vi "获取一个图像区域每一列亮度平均值.vi"(10 "矩形框":dbl[](array[numeric]), 11 "引用句柄输入":T1) -> (3 "数组":dbl[](array[numeric]))   [LabVIEW 2014]
uses:
  <vilib>/vision/Image Controls.llb/IMAQ Image.ctl
  <vilib>/Analysis/baseanly.llb/Mean (DBL).vi
  <vilib>/Analysis/NI_AALBase.lvlib
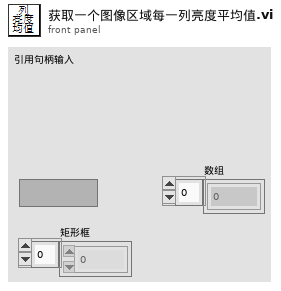
[diagram p1: front panel]
types:
  T1 = typedef "IMAQ Image.ctl" = refnum<image>
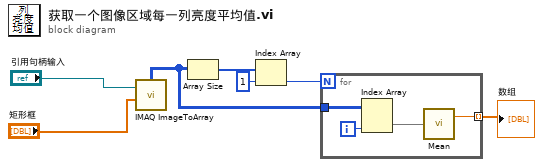
[diagram p0: block diagram]
diagram:
  n1 = call "IMAQ ImageToArray"("Optional Rectangle"="矩形框", "Image"="引用句柄输入") -> ("Image Pixels (U8)"=w1:u8[][])  [unwired: 2 in, 4 out]
  n2 = Array Size(array=w1) -> (size(s)=w2:i32[])
  n3 = Index Array(array=w2, index=1 ("索引")) -> (element=w3:i32)
  n4 = for {
    N: w3 -> [_]
    tunnel: w1 -> [w11]
    tunnel: [w8] -> w5 mode=indexing
    i -> [w10]
    n5 = Index Array(array=w11, index (col)=w10) -> (element=w9:u8[])  [unwired: 1 in]
    n6 = call-poly <vilib>:"Mean.vi"("X"=w9) -> ("mean"=w8:dbl)  [unwired: 1 out]
  }
  "数组" <- w5
